vi "DCMotorClose.vi"(8 "error in":errorcluster, 11 "Device In":u64) -> (0 "error out":errorcluster)   [LabVIEW 2020, in "Phidget DC Motor.lvlib"]
doc: "${DCMotor:CloseHeader}"
uses:
  <instrlib>/Phidgets/Phidget DC Motor/Phidget DC Motor.lvlib
  <instrlib>/Phidgets/Phidget Common/Phidget Common.lvlib
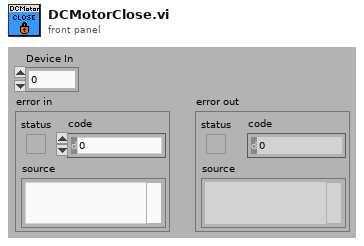
[diagram p1: front panel]
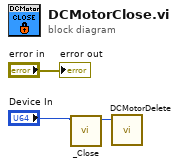
[diagram p0: block diagram]
diagram:
  n1 = call <instrlib>:"_Close.vi"("Device In"="Device In") -> ("Device Out"=w2:u64)  [unwired: 9 in, 1 out]
  n2 = call <instrlib>:"DCMotorDelete.vi"("Device In"=w2) -> ()  [unwired: 10 in, 1 out]
  "error out" <- "error in"
